vi "Pre Launch Init.vi"(11 "Digital Writer in":refnum<class "Digital Writer.lvclass">) -> (0 "error out":errorcluster, 3 "Digital Writer out":refnum<class "Digital Writer.lvclass">)   [LabVIEW 2024, in "DAQmx Actor.lvlib" / "Digital Writer.lvclass"]
doc: "<p>(<strong>Filename</strong>: <span class=\"dnl\">Actor Framework.lvlib:Actor.lvclass:Pre Launch Init.vi</span>)</p>\n<p>Defines behavior that occurs after the <a href=\"nihelplauncher://docs/csh?context=lvcore_lvcomm_af_launch_nested_actor\">Launch Nested Actor</a> method is invoked but before the actor's Actor Core method begins running.</p>\n<p>By default, this method does nothing. A descendant class may override it to define behavior.</p>"
uses:
  Digital Writer.lvclass
  DAQmx Actor/DAQmx Actor.lvclass
  Digital Writer.lvclass/Digital Writer.ctl
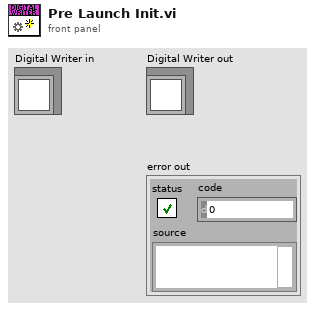
[diagram p1: front panel]
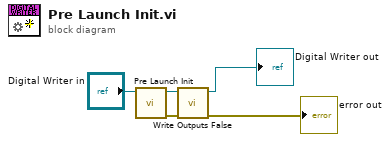
[diagram p0: block diagram]
diagram:
  n1 = call-parent "Pre Launch Init.vi"("DAQmx Actor in"="Digital Writer in") -> ("error out"=w2:errorcluster, "DAQmx Actor out"=w4:refnum<class "Digital Writer.lvclass">)  [unwired: 9 in]
  n2 = call-dynamic "Write Outputs False.vi"("error in (no error)"=w2, "Digital Writer in"=w4) -> ("error out"=→"error out":errorcluster, "Digital Writer out"=→"Digital Writer out":refnum<class "Digital Writer.lvclass">)  [unwired: 8 in]
